vi "mission_select.vi"(1 "Data":dbl) -> (0 "String":string)   [LabVIEW 2017]
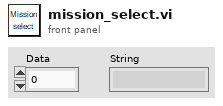
[diagram p1: front panel]
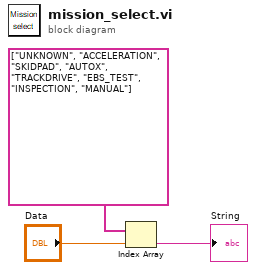
[diagram p0: block diagram]
diagram:
  n1 = Index Array(array=string[] ["UNKNOWN", "ACCELERATION", "SKIDPAD", "AUTOX", "TRACKDRIVE", "EBS_TEST", "INSPECTION", "MANUAL"], index="Data") -> (element=→"String":string)
